vi "ViewPic.vi"(8 "MetaData":string="　This　Picture　is ....", 10 "VarRange":cluster{"Max":dbl, "Min":dbl}, 11 "Data":dbl[][](array[numeric])) -> ()   [LabVIEW 2016]
uses:
  XControls/FalseColorEditer/FalseColorEditer.xctl
  XControls/GradChangeColorBar/GradChangeColorBar.xctl
  <vilib>/picture/picture.llb/imagedata.ctl
panel:
  in  "FalseColorEditer":T1(xcontrol)={"Ratio_R"=[{0.0, 0.0}, {0.5, 1.0}, {1.0, 1.0}], "Ratio_G"=[{0.0, 0.0}, {0.25, 0.0}, {0.75, 1.0}, {1.0, 1.0}], "Ratio_B"=[{0.0, 0.0}, {0.5, 0.0}, {1.0, 1.0}]}
  out "MapTb":T2
  out "Pic":picture
  out "GradChangeColorBar":T3(xcontrol)
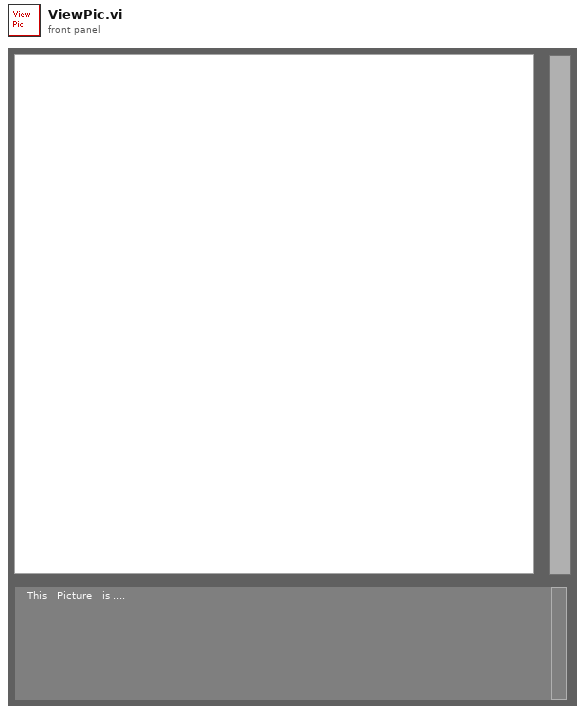
[diagram p1: front panel]
types:
  T1 = cluster{"Ratio_R":cluster{dbl, dbl}[], "Ratio_G":cluster{dbl, dbl}[], "Ratio_B":cluster{dbl, dbl}[]}
  T2 = cluster{"MapVar":dbl[], "RMapTb":cluster{dbl, u8}[], "GMapTb":cluster{dbl, u8}[], "BMapTb":cluster{dbl, u8}[]}
  T3 = cluster{cluster{dbl, "R":dbl}[], cluster{dbl, "G":dbl}[], cluster{dbl, "B":dbl}[]}
  T4 = typedef "imagedata.ctl" = cluster{"image type":i32, "image depth":i32, "image":u8[], "mask":u8[], "colors":u32[], "Rectangle":cluster{"left":i16, "top":i16, "right":i16, "bottom":i16}}
  T5 = typedef "LVBoundsTypeDef.ctl" = cluster{"Width":u32, "Height":u32}
  T6 = cluster{"[0]":i32, "[0]":i32, "[1]":i32, "[0]":i32}
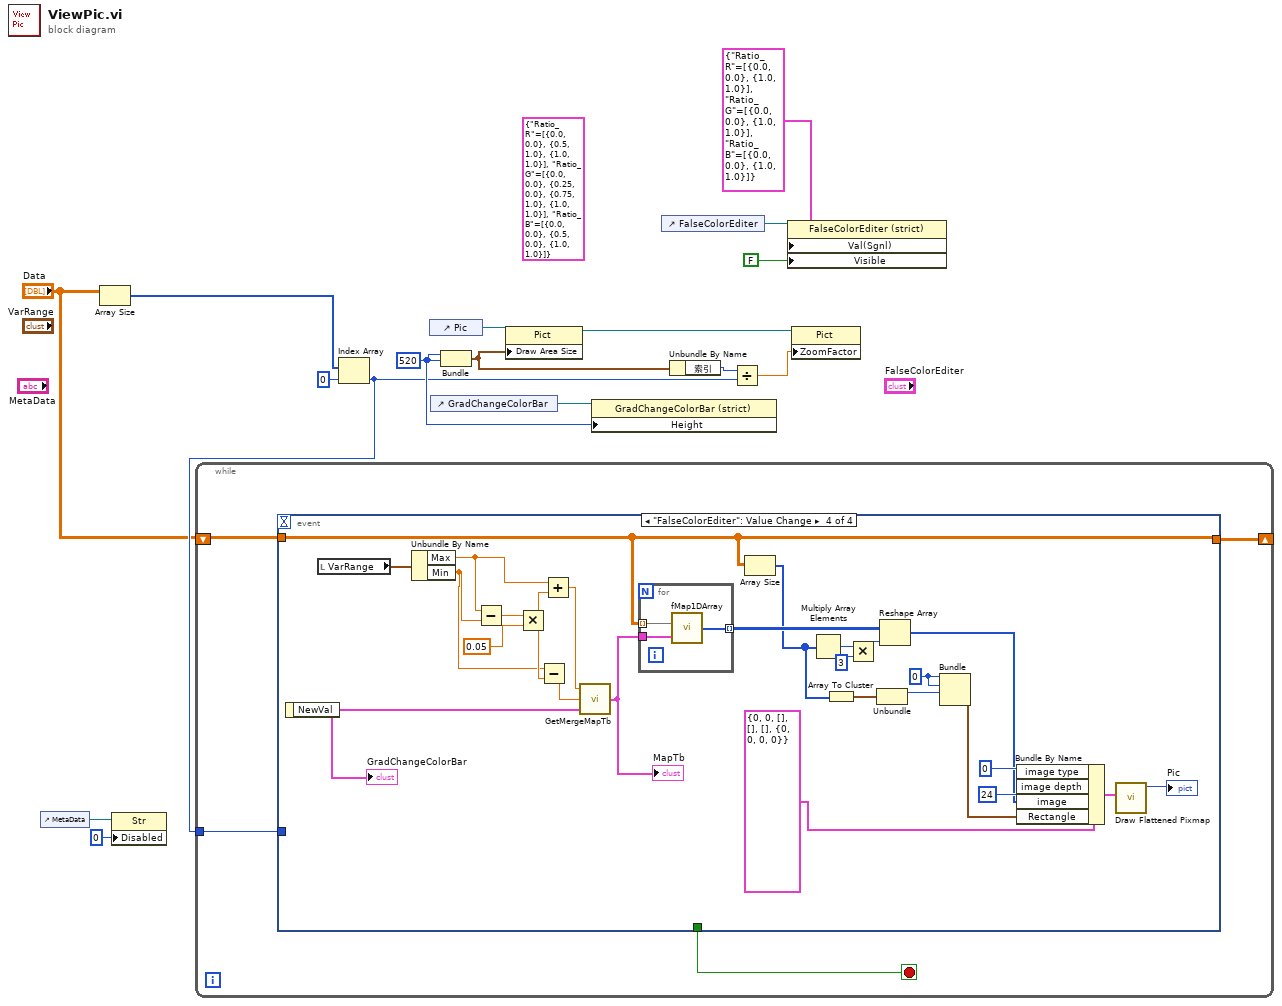
[diagram p0: block diagram]
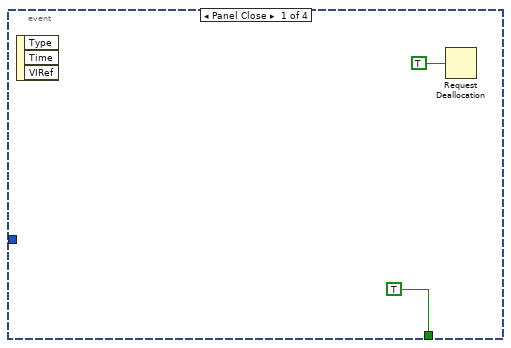
[diagram p2: hidden frame]
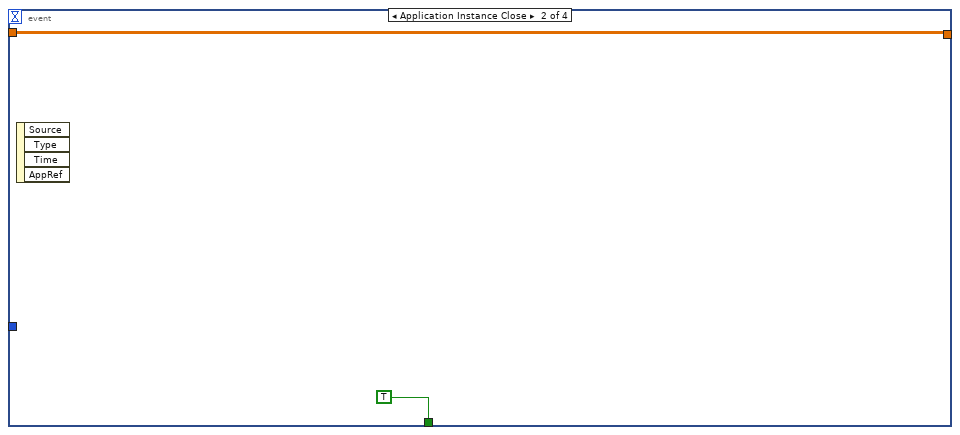
[diagram p3: hidden frame]
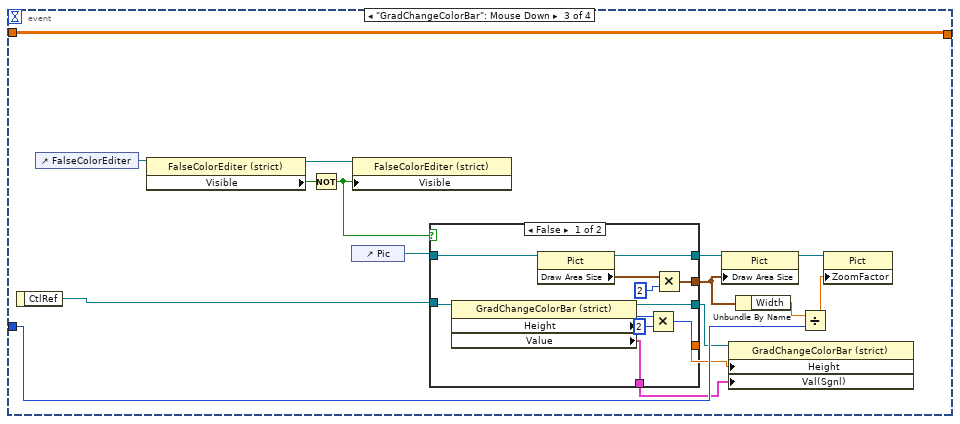
[diagram p4: hidden frame]
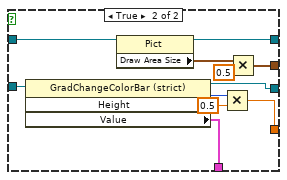
[diagram p5: hidden frame]
diagram:
  w8 = u32 520 ("索引")
  (unwired) T1 {"Ratio_R"=[{0.0, 0.0}, {0.5, 1.0}, {1.0, 1.0}], "Ratio_G"=[{0.0, 0.0}, {0.25, 0.0}, {0.75, 1.0}, {1.0, 1.0}], "Ratio_B"=[{0.0, 0.0}, {0.5, 0.0}, {1.0, 1.0}]} ("新值")
  n1 = control-ref of="MetaData"() -> (w13:refnum<vi>)
  n2 = Array Size(array="Data") -> (size(s)=w15:i32[])
  n3 = property class="Str"(reference=w13, "Disabled"=u8 0 ("禁用")) -> ()  [unwired: 1 in, 2 out]
  n4 = Index Array(array=w15, index=0 ("索引")) -> (element=w3:i32)
  n5 = while {
    tunnel: w3 -> [w20]
    shift-right: [w17] -> _
    shift-left: "Data" -> [w18]
    stop <- w19 stop-if-true
    n6 = event shown="[3] \"FalseColorEditer\": Value Change" {
      selector: _ -> [_ _ _ _]
      dyn-events: _ -> [_ _ _ _]
      timeout: _ -> [_ _ _ _]
      tunnel: [TRUE TRUE _ _] -> w19
      tunnel: w20 -> [_ _ w31 _]
      tunnel: w18 -> [_ w23 w25 w66]
      tunnel: [_ w23 w25 w66] -> w17
      event Panel Close {
        n7 = event-data() -> ()  [unwired: 4 out]
        n8 = Request Deallocation(TRUE ("标志")) -> ()
      }
      event Application Instance Close {
        n9 = event-data() -> ()  [unwired: 5 out]
      }
      event "GradChangeColorBar": Mouse Down {
        n10 = event-data() -> ("CtlRef"=w29:refnum<vi>)  [unwired: 1 out]
        n11 = control-ref of="FalseColorEditer"() -> (w40:refnum<vi>)
        n12 = property class="FalseColorEditer (strict)"(reference=w40) -> (reference out=w39:refnum<vi>, "Visible"=w38:bool)  [unwired: 1 in, 1 out]
        n13 = Not(x=w38) -> (.not. x?=w36:bool)
        n14 = control-ref of="Pic"() -> (w37:refnum<vi>)
        n15 = property class="FalseColorEditer (strict)"(reference=w39, "Visible"=w36) -> ()  [unwired: 1 in, 2 out]
        n16 = case shown="False" w36 {
          tunnel: w37 -> [w51 w62]
          tunnel: [w50 w61] -> w35
          tunnel: [w47 w58] -> w33
          tunnel: w29 -> [w46 w55]
          tunnel: [w45 w54] -> w28
          tunnel: [w42 w53] -> w27
          tunnel: [w41 w52] -> w26
          frame False {
            n17 = property class="GradChangeColorBar (strict)"(reference=w46) -> (reference out=w45:refnum<vi>, "Height"=w44:u32, "Value"=w41:T3)  [unwired: 1 in, 1 out]
            n18 = property class="Pict"(reference=w51) -> (reference out=w50:refnum<vi>, "Draw Area Size"=w49:T5)  [unwired: 1 in, 1 out]
            n19 = Multiply(x=w44, y=u32 2) -> (x*y=w42:u32)
            n20 = Multiply(x=w49, y=u32 2) -> (x*y=w47:T5)
          }
          frame True {
            n21 = property class="GradChangeColorBar (strict)"(reference=w55) -> (reference out=w54:refnum<vi>, "Height"=w56:u32, "Value"=w52:T3)  [unwired: 1 in, 1 out]
            n22 = property class="Pict"(reference=w62) -> (reference out=w61:refnum<vi>, "Draw Area Size"=w59:T5)  [unwired: 1 in, 1 out]
            n23 = Multiply(x=w56, y=sgl 0.5) -> (x*y=w53:sgl)
            n24 = Multiply(x=w59, y=sgl 0.5) -> (x*y=w58:cluster{"Width":sgl, "Height":sgl})
          }
        }
        n25 = property class="Pict"(reference=w35, "Draw Area Size"=w33) -> (reference out=w34:refnum<vi>)  [unwired: 1 in, 1 out]
        n26 = property class="GradChangeColorBar (strict)"(reference=w28, "Height"=w27, "Val(Sgnl)"=w26) -> ()  [unwired: 1 in, 2 out]
        n27 = Unbundle By Name(w33) -> ("Width"=w32:sgl)
        n28 = Divide(x=w32, y=w31) -> (x/y=w30:sgl)
        n29 = property class="Pict"(reference=w34, "ZoomFactor"=w30) -> ()  [unwired: 1 in, 2 out]
      }
      event "FalseColorEditer": Value Change {
        w68 = 0 ("[0]")
        n30 = event-data() -> ("NewVal"=w87:T1)  [unwired: 1 out]
        "GradChangeColorBar" <- w87
        n31 = local read "VarRange"() -> (w89:cluster{"Max":dbl, "Min":dbl})
        n32 = Unbundle By Name(w89) -> ("Max"=w84:dbl, "Min"=w81:dbl)
        n33 = Subtract(x=w84, y=w81) -> (x-y=w86:dbl)
        n34 = Multiply(x=w86, y=0.05) -> (x*y=w82:dbl)
        n35 = Subtract(x=w81, y=w82) -> (x-y=w80:dbl)
        n36 = Add(x=w84, y=w82) -> (x+y=w83:dbl)
        n37 = call "GetMergeMapTb.vi"("FalseColorDat"=w87, "VarRangeMin"=w80, "VarRangeMax"=w83) -> ("MapTb"=w88:T2)
        "MapTb" <- w88
        n38 = for {
          tunnel: w66 -> [w92] mode=indexing
          tunnel: w88 -> [w91]
          tunnel: [w90] -> w73 mode=indexing
          n39 = call "fMap1DArray.vi"("MapTb"=w91, "1DRealVarArray"=w92) -> ("InternalFormatRGBArrForLV"=w90:u8[])
        }
        n40 = Array Size(array=w66) -> (size(s)=w72:i32[])
        n41 = Multiply Array Elements(1:w72) -> (0:w64:i32)
        n42 = Array To Cluster(array=w72) -> (cluster=w71:cluster{"[0]":i32, "[1]":i32})
        n43 = Multiply(x=w64, y=3) -> (x*y=w63:i32)
        n44 = Unbundle(w71) -> ("[0]"=w70:i32, "[1]"=w69:i32)
        n45 = Reshape Array(w73, w63) -> (w76:u8[])
        n46 = Bundle("[0]"=w68, "[0]"=w68, "[1]"=w69, "[0]"=w70) -> (w67:T6)  [unwired: 1 out]
        n47 = Bundle By Name(cluster=T4 {"image type"=0, "image depth"=0, "image"=[], "mask"=[], "colors"=[], "Rectangle"={"left"=0, "top"=0, "right"=0, "bottom"=0}} ("image data"), "image type"=0, "image depth"=24, "image"=w76, "Rectangle"=w67) -> (w75:T4)
        n48 = call <vilib>:"Draw Flattened Pixmap.vi"("image data"=w75) -> ("new picture"=→"Pic":picture)  [unwired: 1 in, 7 out]
      }
    }
  }
  n49 = control-ref of="Pic"() -> (w16:refnum<vi>)
  n50 = control-ref of="GradChangeColorBar"() -> (w9:refnum<vi>)
  n51 = Bundle("索引"=w8, "索引"=w8) -> (w6:cluster{"索引":u32, "索引":u32})  [unwired: 1 out]
  n52 = property class="Pict"(reference=w16, "Draw Area Size"=w6) -> (reference out=w5:refnum<vi>)  [unwired: 1 in, 1 out]
  n53 = property class="GradChangeColorBar (strict)"(reference=w9, "Height"=w8) -> ()  [unwired: 1 in, 2 out]
  n54 = control-ref of="FalseColorEditer"() -> (w11:refnum<vi>)
  n55 = Unbundle By Name(w6) -> ("索引"=w7:u32)
  n56 = Divide(x=w7, y=w3) -> (x/y=w4:dbl)
  n57 = property class="FalseColorEditer (strict)"(reference=w11, "Val(Sgnl)"=T1 {"Ratio_R"=[{0.0, 0.0}, {1.0, 1.0}], "Ratio_G"=[{0.0, 0.0}, {1.0, 1.0}], "Ratio_B"=[{0.0, 0.0}, {1.0, 1.0}]} ("值(信号)"), "Visible"=FALSE ("可见")) -> ()  [unwired: 1 in, 2 out]
  n58 = property class="Pict"(reference=w5, "ZoomFactor"=w4) -> ()  [unwired: 1 in, 2 out]
